vi "upload_from_file.vi"(1 "Spreadsheet path":path) -> (0 "Cell Settings Array 4":T1(array[cluster])=[{"Measure?"=TRUE, "Area (cm^2)"=0.0, "Cell Label"="", "Cell Description"="", "Time between scans (min)"=0.0, "Cell Position"=1, "Scan settings in queue"=0, "Sample holder"=4.0}, {"Measure?"=TRUE, "Area (cm^2)"=0.0, "Cell Label"="", "Cell Description"="", "Time between scans (min)"=0.0, "Cell Position"=2, "Scan settings in queue"=0, "Sample holder"=4.0}, {"Measure?"=TRUE, "Area (cm^2)"=0.0, "Cell Label"="", "Cell Description"="", "Time between scans (min)"=0.0, "Cell Position"=3, "Scan settings in queue"=0, "Sample holder"=4.0}, {"Measure?"=TRUE, "Area (cm^2)"=0.0, "Cell Label"="", "Cell Description"="", "Time between scans (min)"=0.0, "Cell Position"=4, "Scan settings in queue"=0, "Sample holder"=4.0}, {"Measure?"=TRUE, "Area (cm^2)"=0.0, "Cell Label"="", "Cell Description"="", "Time between scans (min)"=0.0, "Cell Position"=5, "Scan settings in queue"=0, "Sample holder"=4.0}, {"Measure?"=TRUE, "Area (cm^2)"=0.0, "Cell Label"="", "Cell Description"="", "Time between scans (min)"=0.0, "Cell Position"=6, "Scan settings in queue"=0, "Sample holder"=4.0}, {"Measure?"=TRUE, "Area (cm^2)"=0.0, "Cell Label"="", "Cell Description"="", "Time between scans (min)"=0.0, "Cell Position"=7, "Scan settings in queue"=0, "Sample holder"=4.0}, {"Measure?"=TRUE, "Area (cm^2)"=0.0, "Cell Label"="", "Cell Description"="", "Time between scans (min)"=0.0, "Cell Position"=8, "Scan settings in queue"=0, "Sample holder"=4.0}, {"Measure?"=TRUE, "Area (cm^2)"=0.0, "Cell Label"="", "Cell Description"="", "Time between scans (min)"=0.0, "Cell Position"=9, "Scan settings in queue"=0, "Sample holder"=4.0}, {"Measure?"=TRUE, "Area (cm^2)"=0.0, "Cell Label"="", "Cell Description"="", "Time between scans (min)"=0.0, "Cell Position"=10, "Scan settings in queue"=0, "Sample holder"=4.0}, {"Measure?"=TRUE, "Area (cm^2)"=0.0, "Cell Label"="", "Cell Description"="", "Time between scans (min)"=0.0, "Cell Position"=11, "Scan settings in queue"=0, "Sample holder"=4.0}, {"Measure?"=TRUE, "Area (cm^2)"=0.0, "Cell Label"="", "Cell Description"="", "Time between scans (min)"=0.0, "Cell Position"=12, "Scan settings in queue"=0, "Sample holder"=4.0}, {"Measure?"=TRUE, "Area (cm^2)"=0.0, "Cell Label"="", "Cell Description"="", "Time between scans (min)"=0.0, "Cell Position"=13, "Scan settings in queue"=0, "Sample holder"=4.0}, {"Measure?"=TRUE, "Area (cm^2)"=0.0, "Cell Label"="", "Cell Description"="", "Time between scans (min)"=0.0, "Cell Position"=14, "Scan settings in queue"=0, "Sample holder"=4.0}, {"Measure?"=TRUE, "Area (cm^2)"=0.0, "Cell Label"="", "Cell Description"="", "Time between scans (min)"=0.0, "Cell Position"=15, "Scan settings in queue"=0, "Sample holder"=4.0}, {"Measure?"=TRUE, "Area (cm^2)"=0.0, "Cell Label"="", "Cell Description"="", "Time between scans (min)"=0.0, "Cell Position"=16, "Scan settings in queue"=0, "Sample holder"=4.0}] {"Scan settings in queue" items=["Regular", "Inverted"]})   [LabVIEW 2011]
uses:
  <vilib>/Utility/file.llb/Read From Spreadsheet File (string).vi
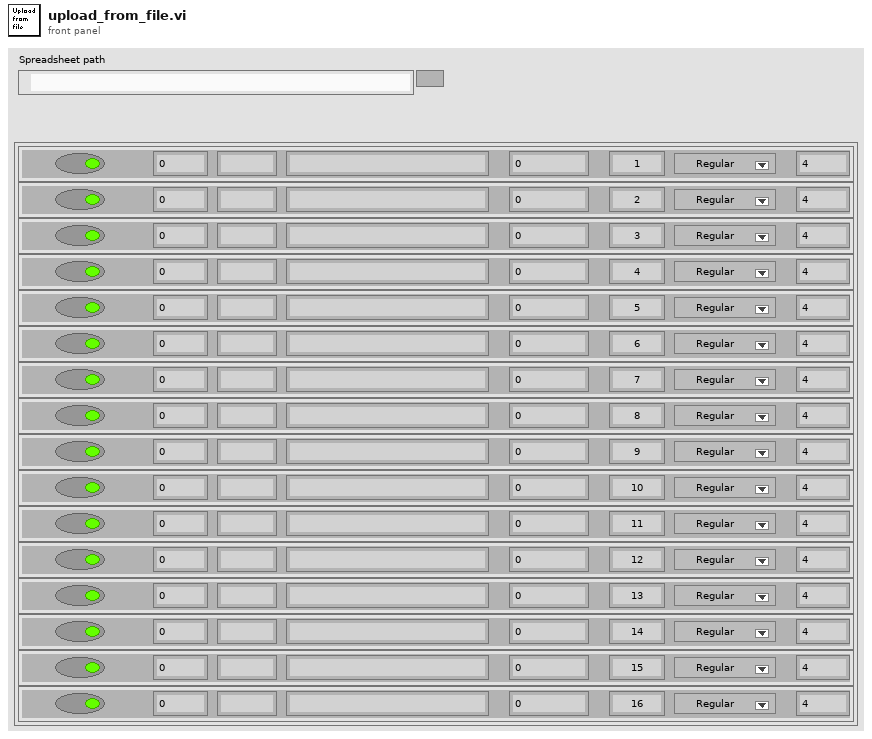
[diagram p1: front panel]
types:
  T1 = cluster{"Measure?":bool, "Area (cm^2)":dbl, "Cell Label":string, "Cell Description":string, "Time between scans (min)":dbl, "Cell Position":i32, "Scan settings in queue":u16, "Sample holder":dbl}[]
  T2 = cluster{"Measure?":bool, "Area (cm^2)":dbl, "Cell Label":string, "Cell Description":string, "Time between scans (min)":dbl, "Cell Position":i32, "Scan settings in queue":u16, "Sample Holder":dbl}
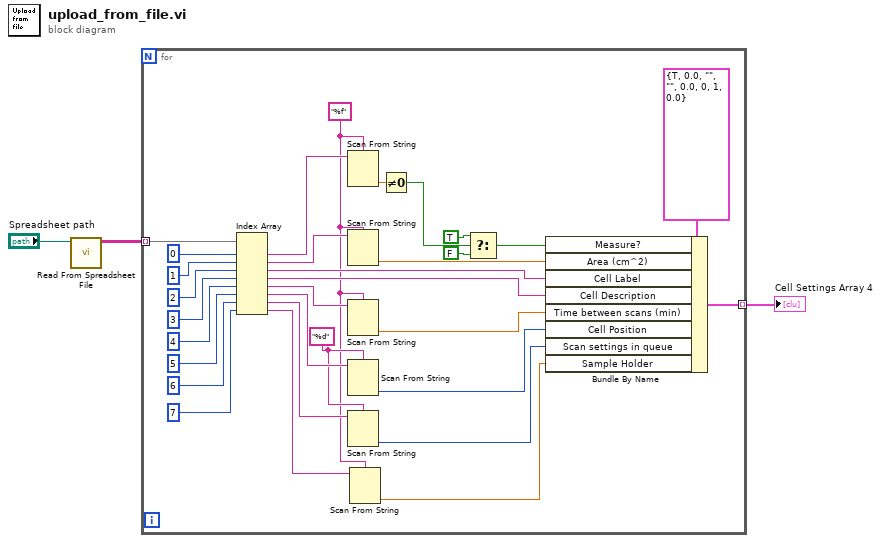
[diagram p0: block diagram]
diagram:
  n1 = call-poly <vilib>:"Read From Spreadsheet File.vi"("file path (dialog if empty)"="Spreadsheet path") -> ("all rows"=w2:string[][])  [unwired: 6 in, 4 out]
  n2 = for {
    tunnel: w2 -> [w34] mode=indexing
    tunnel: [w33] -> w1 mode=indexing
    w7 = "%d" ("format string")
    w6 = "%f" ("format string")
    n3 = Index Array(array=w34, index #1=0 ("index"), index #2=1 ("index"), index #3=2 ("index"), index #4=3 ("index"), index #5=4 ("index"), index #6=5 ("index"), index #7=6 ("index"), index #8=7 ("index")) -> (element #1=w27:string, element #2=w21:string, element #3=w19:string, element #4=w18:string, element #5=w17:string, element #6=w14:string, element #7=w11:string, element #8=w5:string)
    n4 = Scan From String(format string=w6, input string=w27) -> (output 1=w26:dbl)  [unwired: 3 in, 3 out]
    n5 = Scan From String(format string=w6, input string=w21) -> (output 1=w20:dbl)  [unwired: 3 in, 3 out]
    n6 = Scan From String(format string=w6, input string=w17) -> (output 1=w16:dbl)  [unwired: 3 in, 3 out]
    n7 = Scan From String(format string=w7, input string=w14) -> (output 1=w13:i32)  [unwired: 3 in, 3 out]
    n8 = Scan From String(format string=w7, input string=w11) -> (output 1=w9:i32)  [unwired: 3 in, 3 out]
    n9 = Scan From String(format string=w6, input string=w5) -> (output 1=w4:dbl)  [unwired: 3 in, 3 out]
    n10 = Not Equal To 0?(x=w26) -> (x != 0?=w25:bool)
    n11 = Select(t=TRUE, s=w25, f=FALSE) -> (s? t:f=w22:bool)
    n12 = Bundle By Name(cluster=T2 {"Measure?"=TRUE, "Area (cm^2)"=0.0, "Cell Label"="", "Cell Description"="", "Time between scans (min)"=0.0, "Cell Position"=0, "Scan settings in queue"=1, "Sample Holder"=0.0} ("Cluster"), "Measure?"=w22, "Area (cm^2)"=w20, "Cell Label"=w19, "Cell Description"=w18, "Time between scans (min)"=w16, "Cell Position"=w13, "Scan settings in queue"=w9, "Sample Holder"=w4) -> (w33:T2)
  }
  "Cell Settings Array 4" <- w1
